vi "DOTYpeConfig.vi"(0 "object in":refnum<class "AD2_DO_SDK.lvclass">, 2 "DOSingleCh":T1 {"IdleState" items=["PushPull", "OpenDrain", "OpenSource", "TriState"]; "DigitalOutOutput" items=["Pulse", "Custom", "Random"]; "Type" items=["Pulse", "Custom", "Random"]}, 5 "error in (no error)":errorcluster) -> (14 "object out":refnum<class "AD2_DO_SDK.lvclass">, 16 "DOSingleCh Out":T1 {"IdleState" items=["PushPull", "OpenDrain", "OpenSource", "TriState"]; "DigitalOutOutput" items=["Pulse", "Custom", "Random"]; "Type" items=["Pulse", "Custom", "Random"]}, 19 "error out":errorcluster)   [LabVIEW 2021, in "AD2_DO_SDK.lvclass"]
uses:
  AD2_DO_SDK.lvclass
  DOSingleCh.ctl
  AD2_DO_SDK.lvclass/AD2_DO_SDK.ctl
  Olasdwf/Olasdwf.lvlib
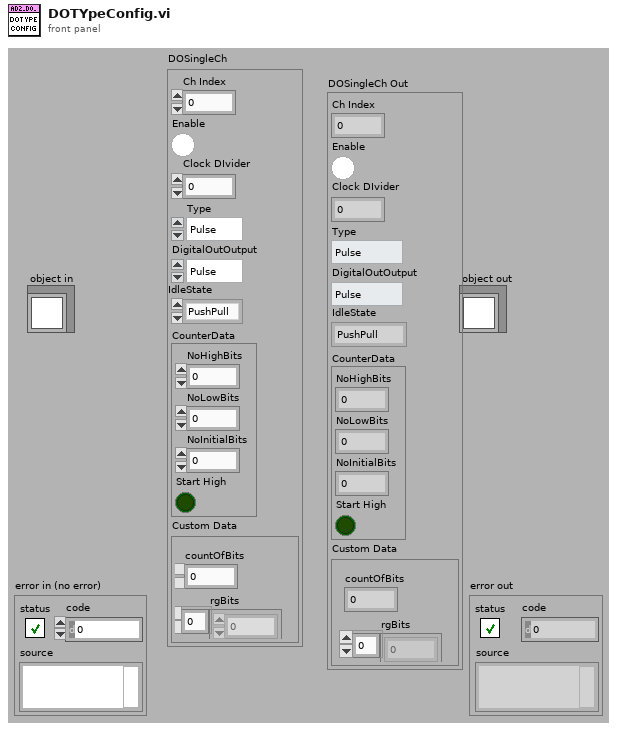
[diagram p1: front panel]
types:
  T1 = typedef "AD2_DO_SDK.lvclass/DOSingleCh.ctl" = cluster{"Ch Index":i32, "Enable":bool, "Clock DIvider":u32, "Type":i32, "DigitalOutOutput":u16, "IdleState":u16, "CounterData":cluster{"NoHighBits":u32, "NoLowBits":u32, "NoInitialBits":u32, "Start High":bool}, "Custom Data":cluster{"countOfBits":u32, "rgBits":u8[]}}
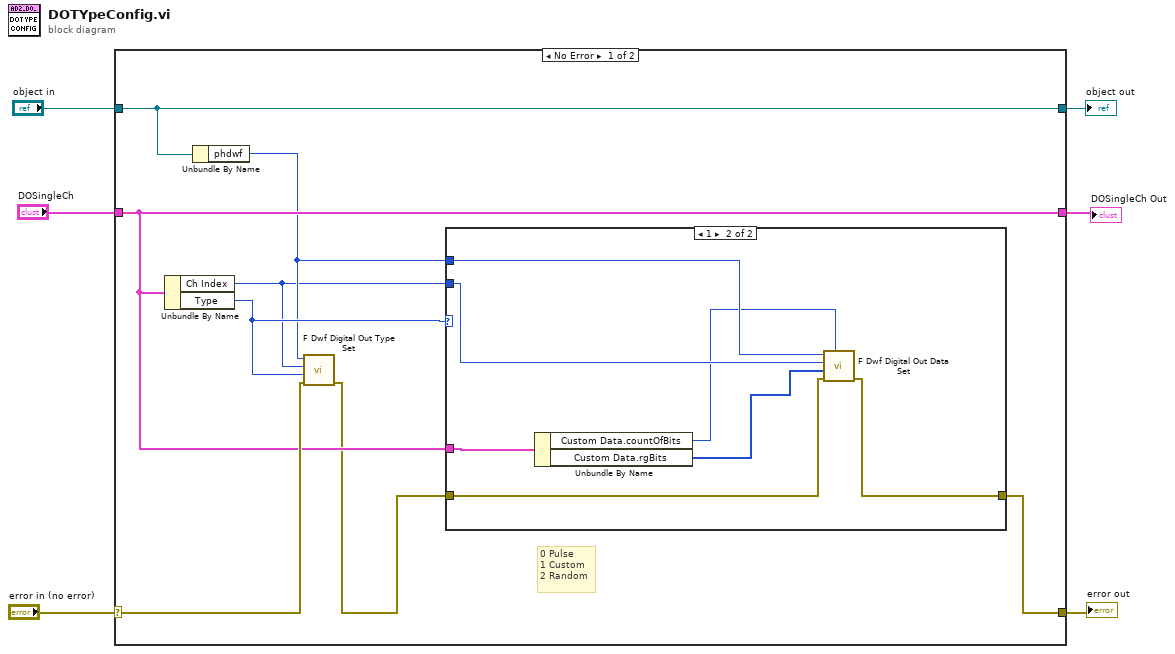
[diagram p0: block diagram]
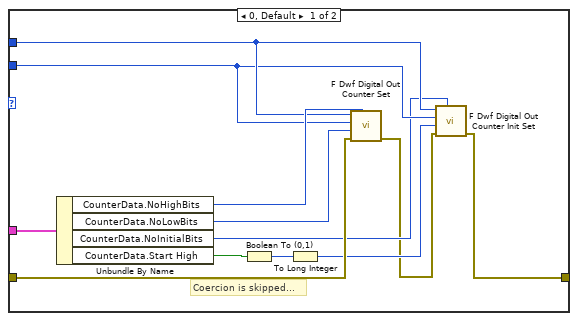
[diagram p2: hidden frame]
diagram:
  n1 = case shown="No Error" "error in (no error)" {
    selector: "error in (no error)" -> [w13 w36]
    tunnel: [w7 w36] -> w5
    tunnel: [w14 w35] -> w3
    tunnel: "object in" -> [w14 w35]
    tunnel: "DOSingleCh" -> [w11 w34]
    tunnel: [w11 w34] -> w1
    frame No Error {
      # "0 Pulse\n1 Custom\n2 Random"
      n2 = Unbundle By Name(w11) -> ("Ch Index"=w9:i32, "Type"=w12:i32)
      n3 = Unbundle By Name(w14) -> ("phdwf"=w10:i32)
      n4 = call "F Dwf Digital Out Type Set.vi"("error in (no error)"=w13, "v"=w12, "idxChannel"=w9, "hdwf"=w10) -> ("error out"=w8:errorcluster)  [unwired: 6 in, 1 out]
      n5 = case shown="1" w12 {
        tunnel: w11 -> [w26 w30]
        tunnel: w10 -> [w22 w33]
        tunnel: w9 -> [w21 w29]
        tunnel: w8 -> [w23 w31]
        tunnel: [w15 w32] -> w7
        frame 0, Default {
          # "Coercion is skipped..."
          n6 = Unbundle By Name(w26) -> ("CounterData.NoHighBits"=w24:u32, "CounterData.NoLowBits"=w25:u32, "CounterData.NoInitialBits"=w17:u32, "CounterData.Start High"=w20:bool)
          n7 = Boolean To (0,1)(Boolean=w20) -> (0, 1=w19:i16)
          n8 = To Long Integer(number=w19) -> (32bit integer=w18:i32)
          n9 = call "F Dwf Digital Out Counter Set.vi"("vHigh"=w24, "error in (no error)"=w23, "vLow"=w25, "idxChannel"=w21, "hdwf"=w22) -> ("error out"=w16:errorcluster)  [unwired: 5 in, 1 out]
          n10 = call "F Dwf Digital Out Counter Init Set.vi"("v"=w17, "error in (no error)"=w16, "fHigh"=w18, "idxChannel"=w21, "hdwf"=w22) -> ("error out"=w15:errorcluster)  [unwired: 5 in, 1 out]
        }
        frame 1 {
          n11 = Unbundle By Name(w30) -> ("Custom Data.countOfBits"=w28:u32, "Custom Data.rgBits"=w27:u8[])
          n12 = call "F Dwf Digital Out Data Set.vi"("countOfBits"=w28, "error in (no error)"=w31, "rgBits"=w27, "idxChannel"=w29, "hdwf"=w33) -> ("error out"=w32:errorcluster)  [unwired: 5 in, 1 out]
        }
      }
    }
    frame Error {
    }
  }
  "error out" <- w5
  "object out" <- w3
  "DOSingleCh Out" <- w1
